vi "Test String Event Type.vi"() -> ()   [LabVIEW 2021]
uses:
  Source/Event Bus/Support/Event Source/Polled_EventSource/Polled_EventSource.lvclass
  C:/TSA/Omni-Bus/Source/Event Bus/Support/Event Source/Event_Source.lvclass
  Source/Omni-Bus/Omni_Bus.lvclass
  Source/Local Bus/Support/Tag List Type.ctl
  <vilib>/Utility/Data Type/Type Definitions/Data Type.ctl
  Source/Local Bus/Local Bus.lvclass
  C:/TSA/Omni-Bus/Source/Omni-Bus/Bus Access/Bus_Access.lvclass
  <vilib>/TSA/Abstract Data Classes/Abs_Types/Type/Abs_Type.lvclass/Abs_Type.ctl
  Source/Omni-Bus/Omni_Bus.lvclass/Omni_Bus.ctl
  Source/Event Bus/Support/Event Type/OnChange/Bool/OnChangeNotifier_Boolean.lvclass/OnChangeNotifier_Boolean.ctl
  Source/Event Bus/Support/Event Source/Event_Source.lvclass/Event_Source.ctl
  Source/Event Bus/Support/Event Source/Polled_EventSource/Polled_EventSource.lvclass/Polled_EventSource.ctl
  Source/Event Bus/Support/Event Type/OnChange/Bool/Properties/Write Data Type.vi
  Source/Event Bus/Support/Event Source/Properties/Write Events.vi
  Source/Event Bus/Support/Event Source/Polled_EventSource/Properties/Write Poll Interval (ms).vi
  Source/Omni-Bus/Support/FindVar.vi
  <vilib>/Utility/error.llb/Clear Errors.vi
  Source/Omni-Bus/Properties/Read Var Map.vi
  <vilib>/TSA/Abstract Data Classes/Abs_Types/Type/Properties/Read Tag.vi
  <vilib>/TSA/Abstract Data Classes/Abs_Types/Boolean/Abs_Boolean.lvclass
  C:/Program Files (x86)/National Instruments/LabVIEW 2021/vi.lib/TSA/Abstract Data Classes/Abs_Types/Type/Abs_Type.lvclass
  <vilib>/TSA/Abstract Data Classes/Abs_Types/Value/Abs_Value.lvclass
  Source/Omni-Bus/Support/Check For Read Only Error.vi
  Source/Omni-Bus/Support/Incorrect Tag String Error.vi
  <vilib>/TSA/Abstract Data Classes/Abs_Types/Type/Abs_Type.lvclass
  <vilib>/Utility/Data Type/NI_Data Type.lvlib
  Source/Event Bus/Support/Event Type/OnChange/String/OnChangeNotifier_String.lvclass
  C:/TSA/Omni-Bus/Source/Local Bus/Local Bus.lvclass
  Source/Omni-Bus/Support/Get/Get String.vi
  C:/Program Files (x86)/National Instruments/LabVIEW 2021/vi.lib/TSA/Abstract Data Classes/Abs_Types/String/Abs_String.lvclass
  C:/Program Files (x86)/National Instruments/LabVIEW 2021/vi.lib/TSA/Abstract Data Classes/Abs_Types/Value/Abs_Value.lvclass
  C:/TSA/Omni-Bus/Source/Event Bus/Support/Event_Polled Type.lvclass
  C:/TSA/Omni-Bus/Source/Event Bus/Support/Event Type/Event_Type.lvclass
  C:/TSA/Omni-Bus/Source/Event Bus/Support/Event Type/OnChange/String/OnChangeNotifier_String.lvclass
  <vilib>/TSA/Abstract Data Classes/Abs_Types/String/Static Write.vi
  <vilib>/TSA/Abstract Data Classes/Abs_Types/String/Abs_String.lvclass
panel:
  out "String":string
  out "Numeric 2":i32
  in  "String 2":string
  out "Timeout":bool
  in  "stop 2":bool
  in  "stop":bool
  out "Numeric":i32
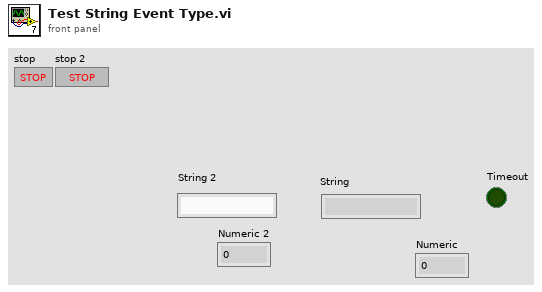
[diagram p1: front panel]
types:
  T1 = typedef "Local Bus.lvclass/Tag List Type.ctl" = cluster{"Tag":string, "Type":T2}
  T2 = typedef "NI_Data Type.lvlib/Data Type.ctl" = enum8{"Invalid Type", "Void", "I8", "I16", "I32", "I64", "U8", "U16", "U32", "U64", "Single Float", "Double Float", "Extended Float", "Single Complex", "Double Complex", "Extended Complex", "Enum U8", "Enum U16", "Enum U32", "Enum U64", "Single Float With Unit", "Double Float With Unit", "Extended Float With Unit", "Single Complex with Unit", "Double Complex with Unit", "Extended Complex with Unit", "Boolean", "String", "Path", "Picture", "Tag", "Array", "Cluster", "Variant", "LV Variant", "Waveform", "Timestamp", "Digital Waveform", "Digital Data", "ExpressData", "Refnum", "External Data", "VI", "Poly VI", "LabVIEW Class Instance", "Fixed Point", "Set Collection", "Map Collection"}
  T3 = typedef "OnChangeNotifier_String.lvclass/Type.ctl" = string
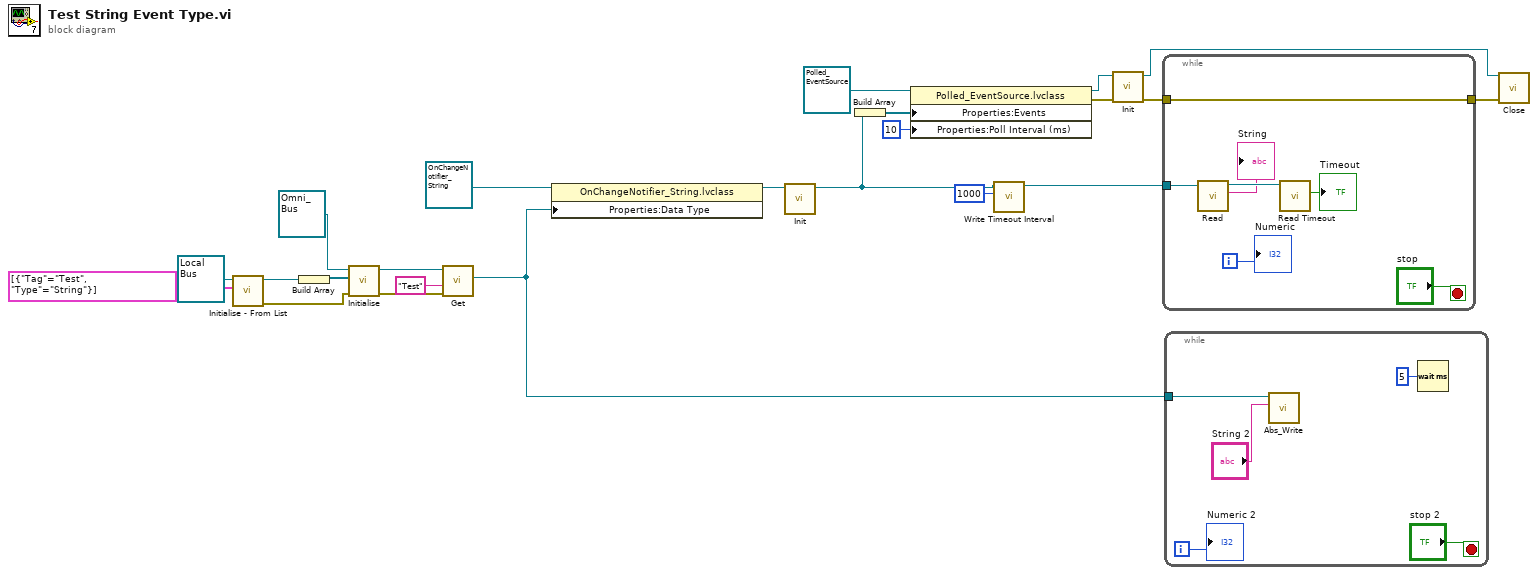
[diagram p0: block diagram]
diagram:
  n1 = call "Initialise - From List.vi"("Tag List"=T1[] [{"Tag"="Test", "Type"=enum."String"}], "Local Bus in"=refnum<class "Local Bus.lvclass"> refnum) -> ("error out"=w16:errorcluster, "Local Bus out"=w18:refnum<class "Local Bus.lvclass">)  [unwired: 8 in]
  n2 = Build Array(w18) -> (w19:refnum<class "Local Bus.lvclass">[])
  n3 = call-dynamic "Initialise.vi"("error in (no error)"=w16, "Bus Access"=w19, "Var Bus in"=refnum<class "Omni_Bus.lvclass"> refnum) -> ("error out"=w21:errorcluster, "Var Bus out"=w22:refnum<class "Omni_Bus.lvclass">)  [unwired: 7 in]
  n4 = call-poly "Get.vi"("error in (no error)"=w21, "Tag"="Test", "Var Bus in"=w22) -> ("Value Out"=w9:refnum<class "Abs_String.lvclass">)  [unwired: 5 in, 3 out]
  n5 = property class="OnChangeNotifier_String.lvclass"(reference=refnum<class "OnChangeNotifier_String.lvclass"> refnum ("OnChangeNotifier_String.lvclass"), "Properties:Data Type"=w9) -> (reference out=w3:refnum<class "OnChangeNotifier_String.lvclass">)  [unwired: 1 in, 1 out]
  n6 = call-dynamic "Init.vi"("Data in"=w3) -> ("Data out"=w2:refnum<class "OnChangeNotifier_String.lvclass">)  [unwired: 9 in, 1 out]
  n7 = Build Array(w2) -> (w15:refnum<class "OnChangeNotifier_String.lvclass">[])
  n8 = property class="Polled_EventSource.lvclass"(reference=refnum<class "Polled_EventSource.lvclass"> refnum ("Polled_EventSource.lvclass"), "Properties:Events"=w15, "Properties:Poll Interval (ms)"=10 ("Poll Interval (ms)")) -> (reference out=w13:refnum<class "Polled_EventSource.lvclass">, error out=w14:errorcluster)  [unwired: 1 in]
  n9 = call-dynamic "Write Timeout Interval.vi"("Timeout Interval (ms)"=1000, "OnChange_Boolean in"=w2) -> ("OnChange_Boolean out"=w8:refnum<class "OnChangeNotifier_String.lvclass">)  [unwired: 8 in, 1 out]
  n10 = call-dynamic "Init.vi"("error in (no error)"=w14, "Data in"=w13) -> ("error out"=w12:errorcluster, "Data out"=w10:refnum<class "Polled_EventSource.lvclass">)  [unwired: 8 in]
  n11 = while {
    tunnel: w8 -> [w27]
    tunnel: w12 -> [w28]
    tunnel: [w28] -> w11
    i -> [w30]
    stop <- "stop" stop-if-true
    n12 = call-dynamic "Read.vi"("String in"=w27) -> ("String"=→"String":T3, "String out"=w26:refnum<class "OnChangeNotifier_String.lvclass">)  [unwired: 8 in, 1 out]
    n13 = call-dynamic "Read Timeout.vi"("OnChange_Boolean in"=w26) -> ("Timeout"=→"Timeout":bool)  [unwired: 8 in, 2 out]
    "Numeric" <- w30
  }
  n14 = while {
    tunnel: w9 -> [w35]
    i -> [w31]
    stop <- "stop 2" stop-if-true
    n15 = call-poly <vilib>:"Abs_Write.vi"("String"="String 2", "Abs_String in"=w35) -> ()  [unwired: 8 in, 2 out]
    n16 = Wait (ms)(milliseconds to wait=u32 5) -> ()  [unwired: 1 out]
    "Numeric 2" <- w31
  }
  n17 = call-dynamic "Close.vi"("error in (no error)"=w11, "Data in"=w10) -> ()  [unwired: 8 in, 2 out]
